vi "ExUtility.vi"(8 "Error In":errorcluster, 11 "Command":string) -> (0 "Error Out":errorcluster, 3 "Response":string)   [LabVIEW 2018]
uses:
  MOKO_LabViewLibrary/MokoLowLevel/MokoLowLovelControl/MLLC_Mode.ctl
  data/ExUtility_PD.ctl
panel:
  in  "Settings":T2
  in  "Error Code":u32
  in  "Utility Name":string="ExUtility"
  in  "Mode":T3
  # "ExUtility"
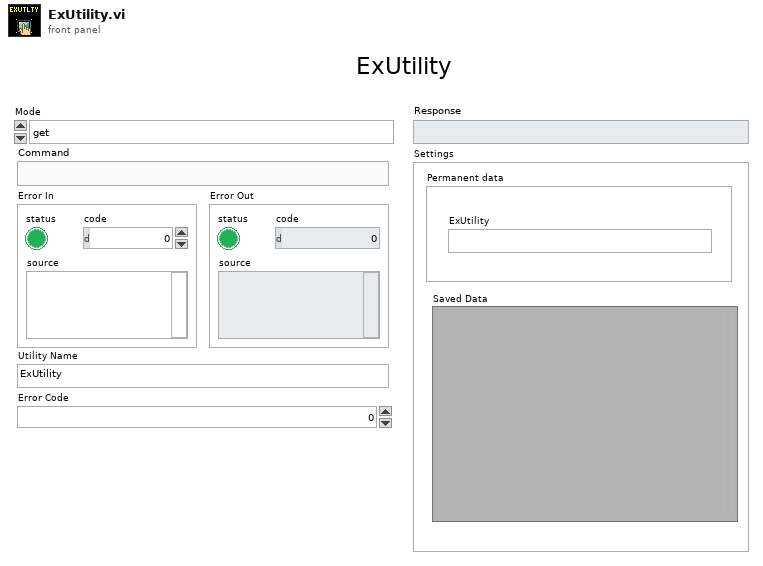
[diagram p1: front panel]
types:
  T1 = typedef "ExUtility_PD.ctl" = cluster{"ExUtility":string}
  T2 = cluster{"Saved Data":variant, "Permanent data":T1}
  T3 = typedef "MLLC_Mode.ctl" = enum16{"get", "set", "close", "Init", "Check"}
  T4 = typedef "MLLC_Error.ctl" = errorcluster
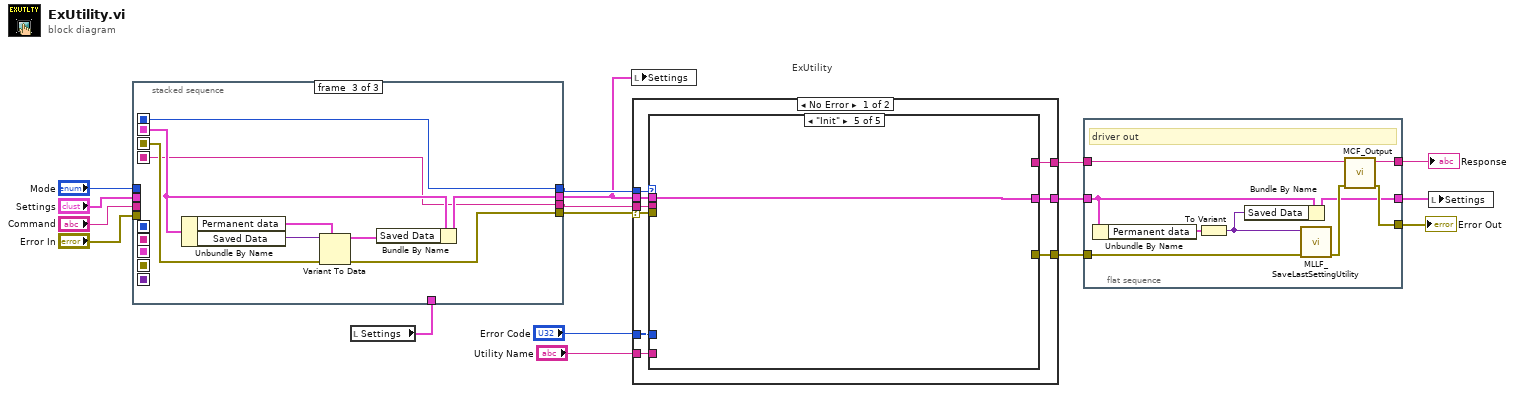
[diagram p0: block diagram]
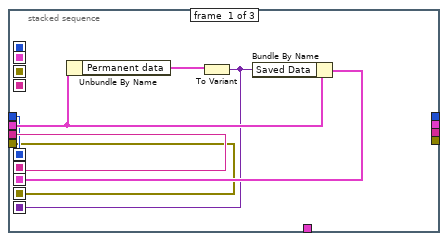
[diagram p2: hidden frame]
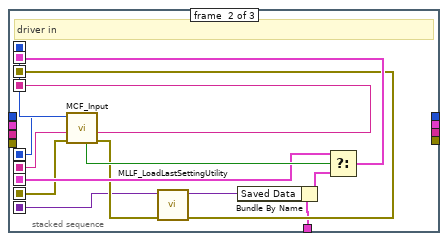
[diagram p3: hidden frame]
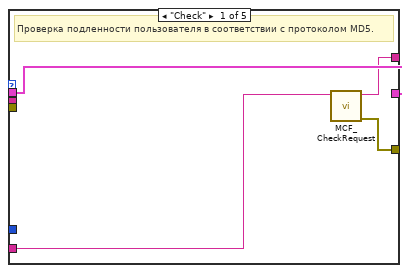
[diagram p4: hidden frame]
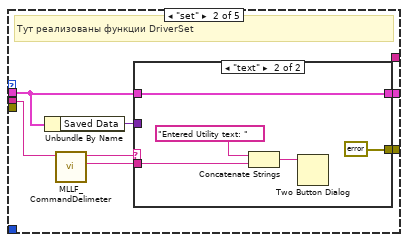
[diagram p5: hidden frame]
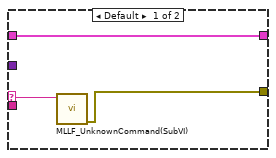
[diagram p6: hidden frame]
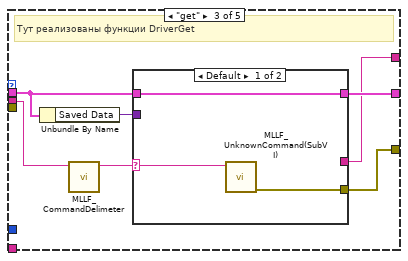
[diagram p7: hidden frame]
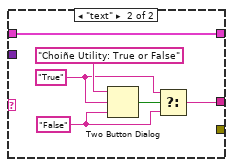
[diagram p8: hidden frame]
diagram:
  # "ExUtility"
  n1 = local read "Settings"() -> (w7:T2)
  n2 = stacked-sequence {
    seq-local: [w21 _ _] -> [_ w36 _]
    seq-local: [w20 _ _] -> [_ w37 _]
    seq-local: [w22 _ _] -> [_ w32 _]
    seq-local: [w19 _ _] -> [_ w31 _]
    seq-local: [w18 _ _] -> [_ w26 _]
    seq-local: [_ w27 _] -> [_ _ w43]
    seq-local: [_ w38 _] -> [_ _ w40]
    seq-local: [_ w35 _] -> [_ _ w39]
    seq-local: [_ w34 _] -> [_ _ w44]
    tunnel: "Command" -> [w21 _ _]
    tunnel: "Mode" -> [w20 _ _]
    tunnel: "Error In" -> [w19 _ _]
    tunnel: "Settings" -> [w23 _ _]
    tunnel: w7 -> [_ w25 _]
    tunnel: [_ _ w39] -> w9
    tunnel: [_ _ w42] -> w10
    tunnel: [_ _ w41] -> w8
    tunnel: [_ _ w40] -> w11
    frame #0 {
      n3 = Unbundle By Name(w23) -> ("Permanent data"=w24:T1)
      n4 = To Variant(anything=w24) -> (Variant=w18:variant)
      n5 = Bundle By Name(cluster=w23, "Saved Data"=w18) -> (w22:T2)
    }
    frame #1 {
      # "driver in"
      n6 = call "MCF_Input.vi"("error in (no error)"=w31, "Command"=w36, "Mode"=w37) -> ("error out"=w30:errorcluster, "Command out"=w35:string, "Mode out"=w38:T3, "Boolean"=w33:bool)  [unwired: 5 in]
      n7 = call "MLLF_LoadLastSettingUtility.vi"("Error In"=w30, "Save data in"=w26) -> ("Error Out"=w27:errorcluster, "Save data out"=w29:variant)  [unwired: 8 in]
      n8 = Bundle By Name(cluster=w25, "Saved Data"=w29) -> (w28:T2)
      n9 = Select(t=w32, s=w33, f=w28) -> (s? t:f=w34:T2)
    }
    frame #2 {
      n10 = Unbundle By Name(w44) -> ("Permanent data"=w45:T1, "Saved Data"=w47:variant)
      n11 = Variant To Data(error in=w43, type=w45, Variant=w47) -> (data=w46:T1, error out=w41:errorcluster)
      n12 = Bundle By Name(cluster=w44, "Saved Data"=w46) -> (w42:T2)
    }
  }
  n13 = local write "Settings"(w10) -> ()
  n14 = case shown="No Error" w8 {
    selector: w8 -> [w52 w95]
    tunnel: [w54 w95] -> w1
    tunnel: w11 -> [w56 _]
    tunnel: [w55 _] -> w6
    tunnel: w9 -> [w53 _]
    tunnel: w10 -> [w49 w94]
    tunnel: "Error Code" -> [w51 _]
    tunnel: "Utility Name" -> [w50 _]
    tunnel: [w48 w94] -> w5
    frame No Error {
      n15 = case shown="\"Init\"" w56 {
        tunnel: [w58 _ w77 _ _] -> w55
        tunnel: [w57 w66 w76 _ _] -> w54
        tunnel: w53 -> [_ w67 w82 _ _]
        tunnel: w52 -> [_ _ _ _ _]
        tunnel: w51 -> [_ _ _ _ _]
        tunnel: w50 -> [w59 _ _ _ _]
        tunnel: w49 -> [w60 w65 w81 w92 w93]
        tunnel: [w60 w64 w80 w92 w93] -> w48
        frame "Check" {
          # "Проверка подленности пользователя в соответствии с протоколом MD5."
          n16 = call "MCF_CheckRequest.vi"("Driver Name"=w59) -> ("Error Out"=w57:errorcluster, "Output String"=w58:string)  [unwired: 9 in]
        }
        frame "set" {
          # "Тут реализованы функции DriverSet"
          n17 = Unbundle By Name(w65) -> ("Saved Data"=w63:variant)
          n18 = call "MLLF_CommandDelimeter.vi"("command with param"=w67) -> ("param 1"=w61:string, "command"=w62:string)  [unwired: 7 in, 2 out]
          n19 = case shown="\"text\"" w62 {
            selector: w62 -> [w69 _]
            tunnel: [w70 w75] -> w64
            tunnel: w65 -> [w70 w75]
            tunnel: w63 -> [_ _]
            tunnel: w61 -> [_ w72]
            tunnel: [w68 errorcluster {"status"=FALSE, "code"=0, "source"=""} ("error IO")] -> w66
            frame Default {
              n20 = call "MLLF_UnknownCommand(SubVI).vi"("Unknown command"=w69) -> ("error out"=w68:errorcluster)  [unwired: 10 in]
            }
            frame "text" {
              n21 = Concatenate Strings("Entered Utility text: ", w72) -> (w71:string)
              n22 = Two Button Dialog(message=w71) -> ()  [unwired: 2 in, 1 out]
            }
          }
        }
        frame "get" {
          # "Тут реализованы функции DriverGet"
          n23 = Unbundle By Name(w81) -> ("Saved Data"=w78:variant)
          n24 = call "MLLF_CommandDelimeter.vi"("command with param"=w82) -> ("command"=w79:string)  [unwired: 7 in, 3 out]
          n25 = case shown="Default" w79 {
            selector: w79 -> [w84 _]
            tunnel: w78 -> [_ _]
            tunnel: w81 -> [w85 w91]
            tunnel: [w85 w91] -> w80
            tunnel: [_ w88] -> w77
            tunnel: [w83 _] -> w76
            frame Default {
              n26 = call "MLLF_UnknownCommand(SubVI).vi"("Unknown command"=w84) -> ("error out"=w83:errorcluster)  [unwired: 10 in]
            }
            frame "text" {
              w86 = "False" ("string")
              w87 = "True" ("string")
              n27 = Two Button Dialog(message="Choiñe Utility: True or False", 1:w86, 2:w87) -> (T button?=w90:bool)
              n28 = Select(t=w87, s=w90, f=w86) -> (s? t:f=w88:string)
            }
          }
        }
        frame "close" {
        }
        frame "Init" {
        }
      }
    }
    frame Error {
    }
  }
  n29 = flat-sequence {
    tunnel: [w104] -> w4
    tunnel: [w103] -> w2
    tunnel: w6 -> [w102]
    tunnel: w1 -> [w101]
    tunnel: w5 -> [w97]
    tunnel: [w99] -> w3
    frame #0 {
      # "driver out"
      n30 = Unbundle By Name(w97) -> ("Permanent data"=w96:T1)
      n31 = To Variant(anything=w96) -> (Variant=w98:variant)
      n32 = Bundle By Name(cluster=w97, "Saved Data"=w98) -> (w99:T2)
      n33 = call "MLLF_SaveLastSettingUtility.vi"("error in"=w101, "Saved Data"=w98) -> ("error out"=w100:T4)  [unwired: 8 in, 1 out]
      n34 = call "MCF_Output.vi"("Error In"=w100, "Input"=w102) -> ("Error Out"=w103:errorcluster, "Output"=w104:string)  [unwired: 8 in]
    }
  }
  n35 = local write "Settings"(w3) -> ()
  "Response" <- w4
  "Error Out" <- w2
